vi "Set Cookie Instance.vi"(8 "error in (no error)":errorcluster, 10 "Cookie":refnum<class "Cookie.lvclass">, 11 "Response in":refnum<class "Response.lvclass">) -> (0 "error out":errorcluster, 3 "Response out":refnum<class "Response.lvclass">)   [LabVIEW 2020, in "HTTP Utils.lvlib" / "Response.lvclass"]
doc: "Adds a Set-Cookie header to the response using a Cookie class instance. Cookie names must be unique."
uses:
  Response.lvclass
  Response.lvclass/Response.ctl
  Cookie/Cookie.lvclass
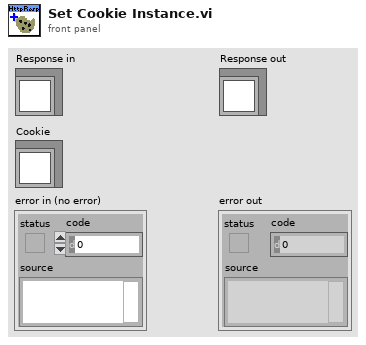
[diagram p1: front panel]
types:
  T1 = typedef "HTTP Utils.lvlib/Cookie Map.ctl" = map{string, refnum<class "Cookie.lvclass">}
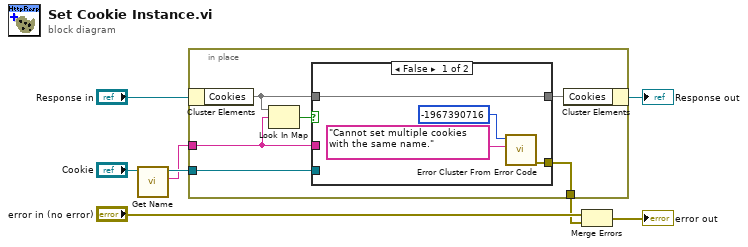
[diagram p0: block diagram]
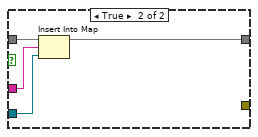
[diagram p2: hidden frame]
diagram:
  n1 = call "Get Name.vi"("Cookie in"="Cookie") -> ("Name"=w4:string, "Cookie out"=w5:refnum<class "Cookie.lvclass">)  [unwired: 8 in, 1 out]
  n2 = in-place {
    in-place-border: w5 -> [w13]
    in-place-border: w4 -> [w11]
    in-place-border: [w9] -> w1
    n3 = in-place-cluster #1("Response in") -> ("Cookies"=w14:T1)
    n4 = Look In Map(map=w14, key=w11) -> (key not found?=w12:bool)  [unwired: 1 in, 1 out]
    n5 = case shown="False" w12 {
      tunnel: w14 -> [w18 w22]
      tunnel: w13 -> [_ w20]
      tunnel: w11 -> [_ w21]
      tunnel: [w18 w19] -> w10
      tunnel: [w15 _] -> w9
      frame False {
        n6 = call <vilib>:"Error Cluster From Error Code.vi"("error message (\"\")"="Cannot set multiple cookies with the same name." ("error message (\"\")"), "error code (0)"=-1967390716) -> ("error out"=w15:errorcluster)  [unwired: 7 in]
      }
      frame True {
        n7 = Insert Into Map(map in=w22, key=w21, value=w20) -> (map out=w19:T1)  [unwired: 2 out]
      }
    }
    n8 = in-place-cluster #1("Cookies"=w10) -> (→"Response out":refnum<class "Response.lvclass">)
  }
  n9 = Merge Errors("error in (no error)", w1) -> (→"error out":errorcluster)
